vi "WC_Drive_Vbus_DriveMotors.vi"(8 "Error":errorcluster, 9 "RightSpeed":dbl, 10 "LeftSpeed":dbl, 11 "RobotDriveDevRef":T1={"DevStatus"={"status"=FALSE, "code"=0, "source"=""}, "Motors[]"=[], "Square Inputs"=FALSE, "Max Output"=1.0}) -> (0 "Error Out":errorcluster, 3 "RobotDriveDevRef Out":T1={"DevStatus"={"status"=FALSE, "code"=0, "source"=""}, "Motors[]"=[], "Square Inputs"=FALSE, "Max Output"=1.0})   [LabVIEW 2017]
doc: "Determines the motor configuration and sends the speed values to the appropriate motors.\n\nThis software is licensed. Open the labview\\readme\\WPI Robotics Library Open Source License.txt file for more information."
uses:
  <vilib>/Rock Robotics/WPI/RobotDrive/WPI_RobotDriveDevRef.ctl
  <vilib>/Rock Robotics/WPI/MotorControl/WPI_MotorControlDeviceRef.ctl
  <vilib>/Rock Robotics/WPI/MotorControl/WPI_MotorControlType.ctl
  <vilib>/Rock Robotics/SystemInterfaces/DIO/FPGA_DIOPWMChannel.ctl
  <vilib>/Rock Robotics/WPI/PWM/WPI_PWMDeadband.ctl
  <vilib>/Rock Robotics/SystemInterfaces/DIO/FPGA_DIOChannel.ctl
  System Drivers/Phoenix-LabVIEW/Motor Controller/Controls/CTRE_Phoenix_MotorControl_ControlMode.ctl
  _SHARE ALL/RoboRio Share All/SRX Share All/TypeDefs SRX/Cluster_SRX_Mode and Value.ctl
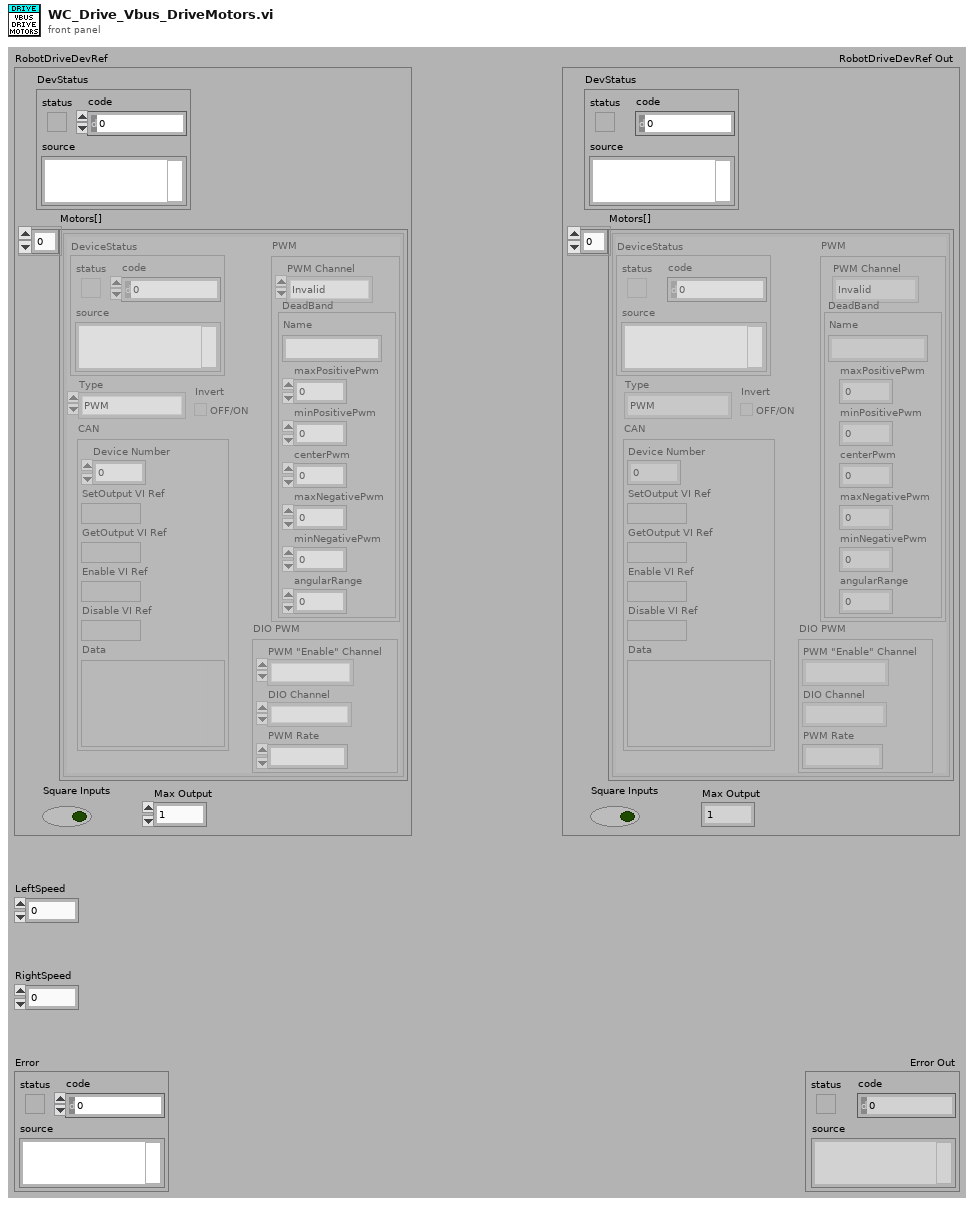
[diagram p1: front panel]
types:
  T1 = typedef "WPI_RobotDriveDevRef.ctl" = cluster{"DevStatus":errorcluster, "Motors[]":T2[], "Square Inputs":bool, "Max Output":dbl}
  T2 = typedef "WPI_MotorControlDeviceRef.ctl" = cluster{"DeviceStatus":errorcluster, "Type":T3, "PWM":cluster{"PWM Channel":T4, "DeadBand":T5}, "CAN":cluster{"Device Number":u8, "SetOutput VI Ref":variant, "GetOutput VI Ref":variant, "Enable VI Ref":variant, "Disable VI Ref":variant, "Data":variant}, "Invert":bool, "DIO PWM":cluster{"PWM \"Enable\" Channel":T4, "DIOChannel":T6, "PWM Rate":dbl}}
  T3 = typedef "WPI_MotorControlType.ctl" = enum16{"PWM", "CAN", "DIO PWM"}
  T4 = typedef "FPGA_DIOPWMChannel.ctl" = enum8{"PWM 0", "PWM 1", "PWM 2", "PWM 3", "PWM 4", "PWM 5", "PWM 6", "PWM 7", "PWM 8", "PWM 9", "PWM MXP 0", "PWM MXP 1", "PWM MXP 2", "PWM MXP 3", "PWM MXP 4", "PWM MXP 5", "PWM MXP 6", "PWM MXP 7", "PWM MXP 8", "PWM MXP 9", "Invalid"}
  T5 = typedef "WPI_PWMDeadband.ctl" = cluster{"Name":string, "maxPositivePwm":i32, "minPositivePwm":i32, "centerPwm":i32, "maxNegativePwm":i32, "minNegativePwm":i32, "angularRange":u16}
  T6 = typedef "FPGA_DIOChannel.ctl" = enum8{"DIO 0", "DIO 1", "DIO 2", "DIO 3", "DIO 4", "DIO 5", "DIO 6", "DIO 7", "DIO 8", "DIO 9", "DIO MXP 0", "DIO MXP 1", "DIO MXP 2", "DIO MXP 3", "DIO MXP 4", "DIO MXP 5", "DIO MXP 6", "DIO MXP 7", "DIO MXP 8", "DIO MXP 9", "DIO MXP 10", "DIO MXP 11", "DIO MXP 12", "DIO MXP 13", "DIO MXP 14", "DIO MXP 15", "SPI Port CS1", "SPI Port CS2", "SPI Port CS3", "SPI Port MISO", "SPI Port MOSI", "Invalid"}
  T7 = typedef "Cluster_SRX_Mode and Value.ctl" = cluster{"Mode":T8, "Value":dbl}
  T8 = typedef "CTRE_Phoenix_MotorControl_ControlMode.ctl" = u16
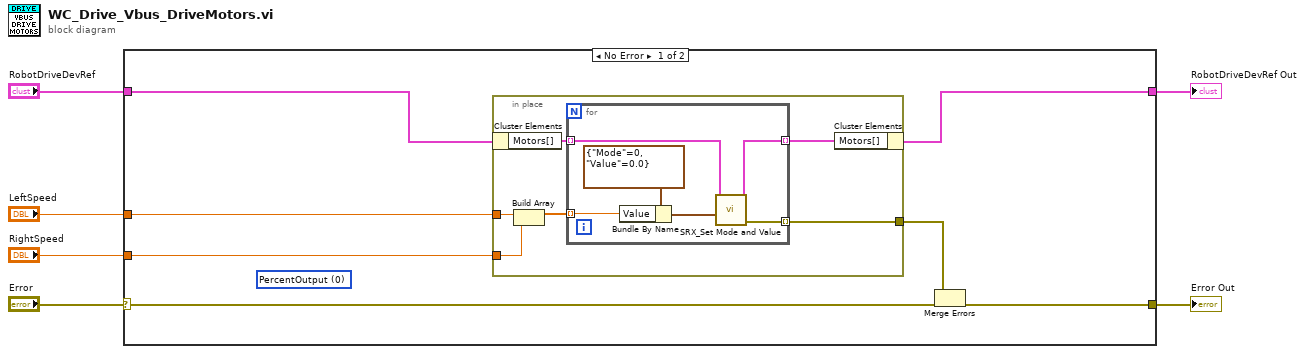
[diagram p0: block diagram]
diagram:
  n1 = case shown="No Error" "Error" {
    selector: "Error" -> [w8 w27]
    tunnel: "RobotDriveDevRef" -> [w13 w26]
    tunnel: [w7 w26] -> w5
    tunnel: "LeftSpeed" -> [w12 _]
    tunnel: "RightSpeed" -> [w11 _]
    tunnel: [w10 w27] -> w1
    frame No Error {
      (unwired) T8 0 items=["PercentOutput"=0, "Position"=1, "Velocity"=2, "Current"=3, "Follower"=5, "MotionProfile"=6, "MotionMagic"=7, "MotionMagicArc"=8, "MotionProfileArc"=10, "Disabled"=15] ("Control Mode")
      n2 = in-place {
        in-place-border: [w19] -> w9
        in-place-border: w12 -> [w16]
        in-place-border: w11 -> [w15]
        n3 = in-place-cluster #1(w13) -> ("Motors[]"=w18:T2[])
        n4 = Build Array(w16, w15) -> (w14:dbl[])
        n5 = for {
          tunnel: [w25] -> w19 mode=indexing
          tunnel: w18 -> [w24] mode=indexing
          tunnel: [w23] -> w17 mode=indexing
          tunnel: w14 -> [w20] mode=indexing
          n6 = Bundle By Name(cluster=T7 {"Mode"=0, "Value"=0.0} ("Mode And Value"), "Value"=w20) -> (w21:T7)
          n7 = call "SRX_Set Mode and Value.vi"("Mode And Value"=w21, "PhoenixMotorControlDevRef"=w24) -> ("Error Out"=w25:errorcluster, "PhoenixMotorControlDevRef Out"=w23:T2)  [unwired: 8 in]
        }
        n8 = in-place-cluster #1("Motors[]"=w17) -> (w7:T1)
      }
      n9 = Merge Errors(w9, w8) -> (w10:errorcluster)
    }
    frame Error {
    }
  }
  "RobotDriveDevRef Out" <- w5
  "Error Out" <- w1
